vi "PSU interface to use GFV.vi"(1 "Action":enum16{"Get", "Set"}(ring), 7 "PSU type Inn in":T1, 11 "error in (no error)":errorcluster) -> (8 "PSU type  out":T1, 15 "error out":errorcluster)   [LabVIEW 2011]
uses:
  PCP interface/PSU Type.ctl
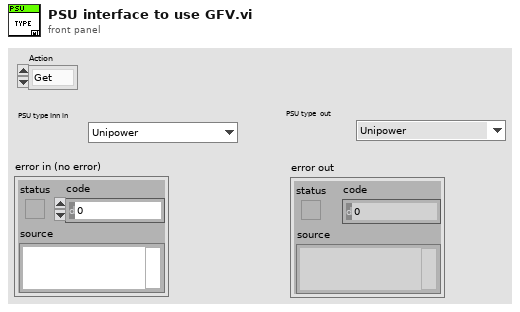
[diagram p1: front panel]
types:
  T1 = typedef "PSU Type.ctl" = enum16{"Unipower", "Magna 8.3A", "Magna 12A", "None"}
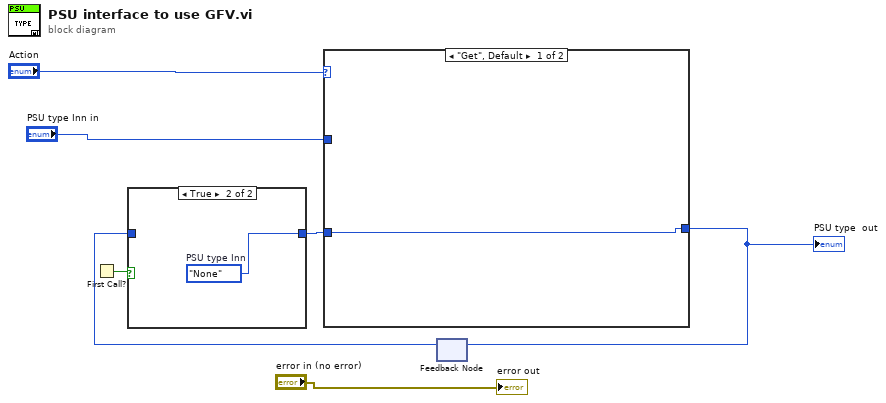
[diagram p0: block diagram]
diagram:
  n1 = First Call?() -> (First Call?: T/F=w2:bool)
  n2 = feedback #1() -> (w7:T1)  [unwired: 1 in]
  n3 = case shown="True" w2 {
    tunnel: [w8 w9] -> w6
    tunnel: w7 -> [w8 _]
    frame False {
    }
    frame True {
      w9 = PSU_Type."None"  # PSU type Inn
    }
  }
  n4 = case shown="\"Get\", Default" "Action" {
    tunnel: "PSU type Inn in" -> [_ w11]
    tunnel: [w10 w11] -> w5
    tunnel: w6 -> [w10 _]
    frame "Get", Default {
    }
    frame "Set" {
    }
  }
  "PSU type  out" <- w5
  n5 = feedback-in #1(w5) -> ()
  "error out" <- "error in (no error)"
